vi "Image_Standardize_Per_Channel.vi"(11 "Input 3D":sgl[][][](array[numeric])) -> (3 "Normalized":sgl[][][](array[numeric]))   [LabVIEW 2020]
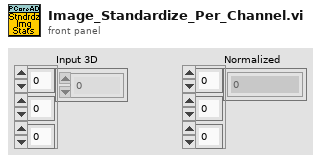
[diagram p1: front panel]
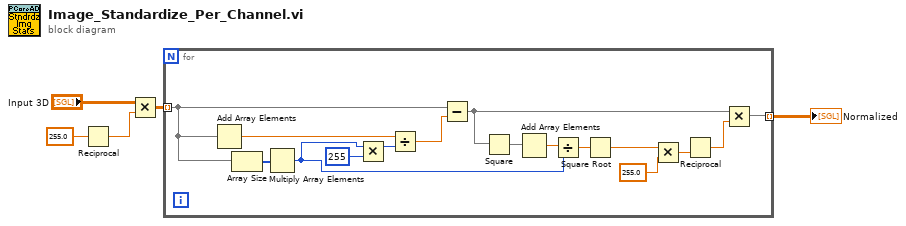
[diagram p0: block diagram]
diagram:
  n1 = Reciprocal(x=sgl 255.0 ("R")) -> (1/x=w4:sgl)
  n2 = Multiply(x="Input 3D", y=w4) -> (x*y=w2:sgl[][][])
  n3 = for {
    tunnel: w2 -> [w21] mode=indexing
    tunnel: [w10] -> w1 mode=indexing
    n4 = Add Array Elements(numeric array=w21) -> (sum=w20:sgl)
    n5 = Array Size(array=w21) -> (size(s)=w19:i32[])
    n6 = Multiply Array Elements(1:w19) -> (0:w15:i32)
    n7 = Multiply(x=w15, y=255) -> (x*y=w7:i32)
    n8 = Divide(x=w20, y=w7) -> (x/y=w18:sgl)
    n9 = Subtract(x=w21, y=w18) -> (x-y=w12:sgl[][])
    n10 = Square(x=w12) -> (x^2=w17:sgl[][])
    n11 = Add Array Elements(numeric array=w17) -> (sum=w16:sgl)
    n12 = Divide(x=w16, y=w15) -> (x/y=w14:sgl)
    n13 = Square Root(x=w14) -> (sqrt(x)=w11:sgl)
    n14 = Multiply(x=w11, y=sgl 255.0) -> (x*y=w9:sgl)
    n15 = Reciprocal(x=w9) -> (1/x=w13:sgl)
    n16 = Multiply(x=w12, y=w13) -> (x*y=w10:sgl[][])
  }
  "Normalized" <- w1
